vi "test_vision.vi"() -> ()   [LabVIEW 2011]
uses:
  <vilib>/vision/NI_Vision_Development_Module.lvlib
panel:
  out "Exe Times":u32[](array[numeric])
  out "Total Execution Time":u32
  out "Avg Execution Time":dbl
  in  "Range":cluster{"Lower value":sgl, "Upper value":sgl}={"Lower value"=218.04347, "Upper value"=255.0} {"Lower value" scale=0.0..255.0; "Upper value" scale=0.0..255.0}
  in  "Score Limits":T1={"Rect Coverage"=76.0, "Aspect Ratio"=0.0, "X Edge Strength"=40.0, "Y Edge Strength"=50.0}
  in  "Area Size Limit":i32=444
  in  "Particle Count Limit":i32=8
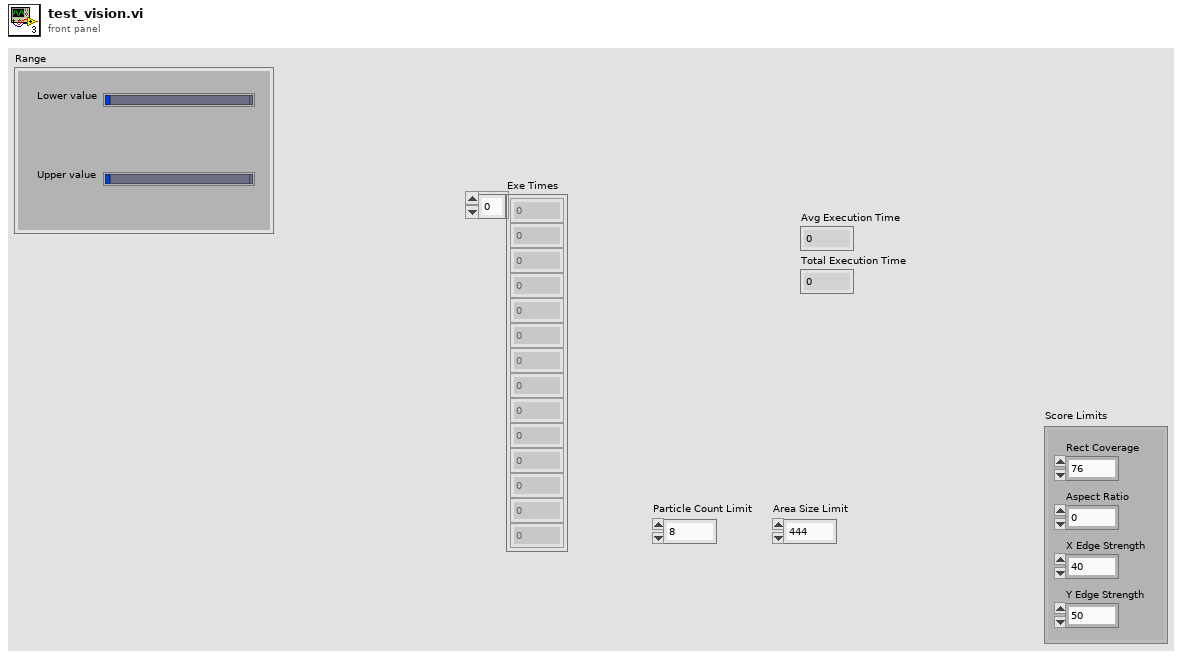
[diagram p1: front panel]
types:
  T1 = cluster{"Rect Coverage":dbl, "Aspect Ratio":dbl, "X Edge Strength":dbl, "Y Edge Strength":dbl}
  T2 = typedef "Image Type" = u32
  T3 = typedef "IMAQ Image.ctl" = refnum<image>
  T4 = enum32{"AutoM", "Close", "Dilate", "Erode", "Gradient", "Gradient in", "Gradient out", "HitMiss", "Open", "PClose", "POpen", "Thick", "Thin"}
  T5 = enum32{"AutoM", "Close", "Dilate", "Erode", "Gradient", "Gradient out", "Gradient in", "Hit miss", "Open", "PClose", "POpen", "Thick", "Thin"}
  T6 = cluster{cluster{"Left":dbl, "Top":dbl, "Right":dbl, "Bottom":dbl}, cluster{"Score":dbl, "Score":dbl, "X Score":dbl, "Y Score":dbl}, "Clipped Edge":cluster{"Left":bool, "Top":bool, "Right":bool, "Bottom":bool}}[]
  T7 = typedef "Camera State.ctl" = enum16{"No Targets", "Low Confidence", "Medium Confidence", "High Confidence", "Camera Error"}
  T8 = cluster{"X Position":dbl, "Distance":dbl, "Camera State":T7}
  T9 = typedef "Diamond Target Output.ctl" = cluster{"Position":cluster{"X":dbl, "Y":dbl, "Distance":dbl}, "Est. Position":T10, "Target Confidence":T11}
  T10 = typedef "Rectangle Position.ctl" = enum16{"Unknown", "Top", "Right", "Left", "Bottom"}
  T11 = typedef "Target Confidence.ctl" = enum16{"Good", "Good-Clipped Y", "Marginal-Clipped X"}
  T12 = typedef "Line.ctl" = cluster{"First Point":cluster{"X":dbl, "Y":dbl, "Index":dbl}, "Second Point":cluster{"X":dbl, "Y":dbl, "Index":dbl}, "theta":dbl, "Direction":T13, "Line Confidence":T14}
  T13 = typedef "Direction.ctl" = enum16{"Rt", "Rt-Up", "Up", "Lt-Up", "Lt", "Lt-Dn", "Dn", "Rt-Dn", "Unknown"}
  T14 = typedef "Line Confidence.ctl" = enum16{"Good", "Bad"}
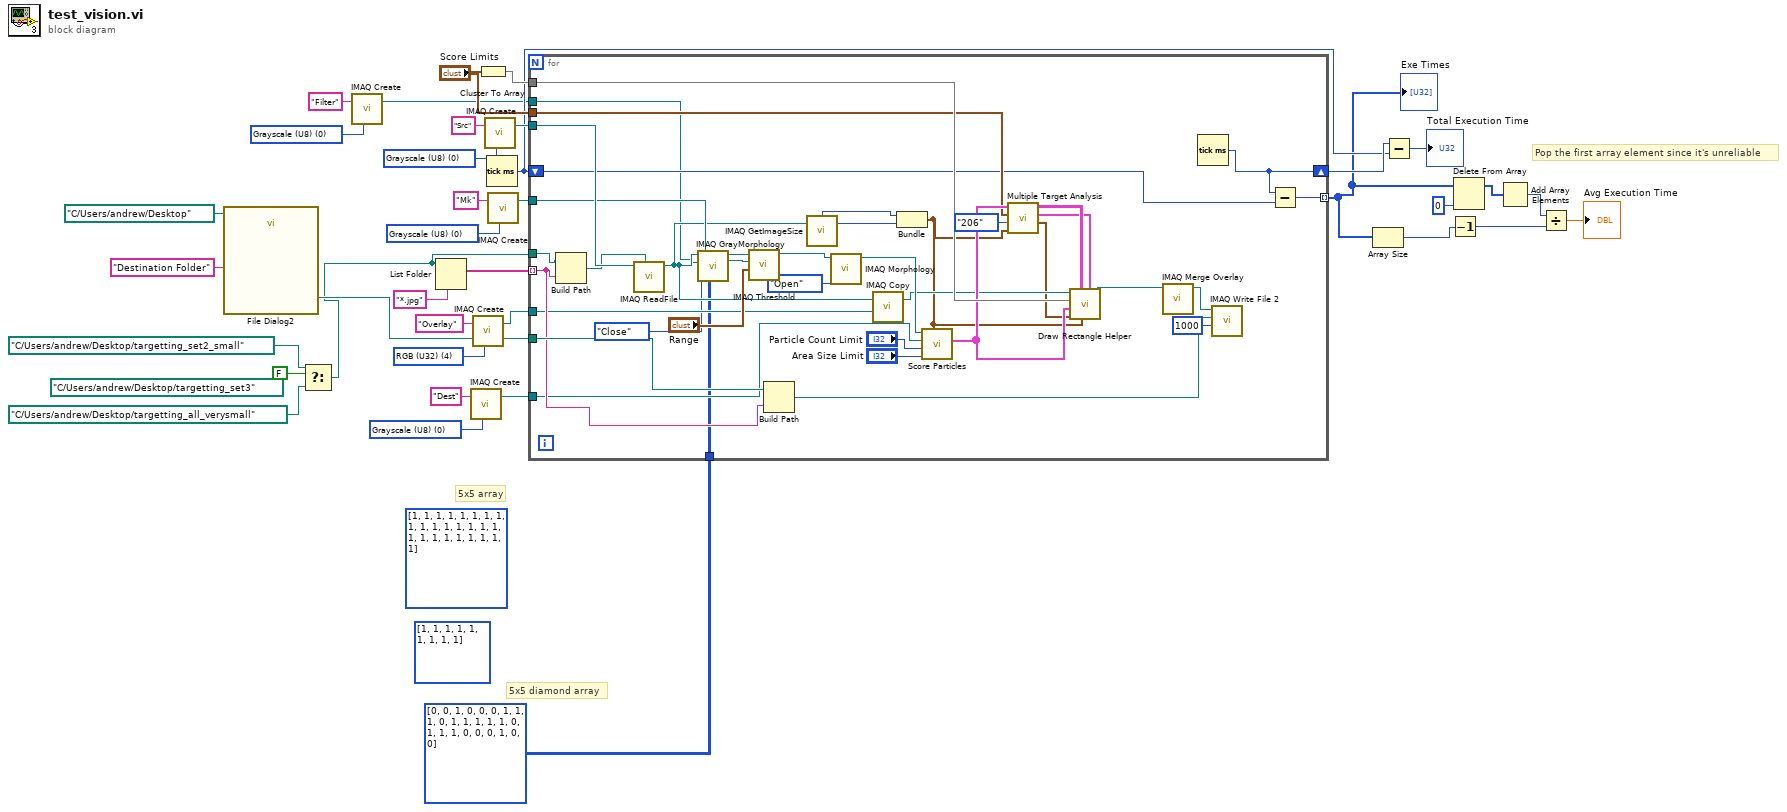
[diagram p0: block diagram]
diagram:
  (unwired) i32[][] [[1, 1, 1], [1, 1, 1], [1, 1, 1]] ("Structuring Element")
  (unwired) i32[][] [[1, 1, 1, 1, 1], [1, 1, 1, 1, 1], [1, 1, 1, 1, 1], [1, 1, 1, 1, 1], [1, 1, 1, 1, 1]] ("Structuring Element")
  w4 = T2 0 items=["Grayscale (U8)", "Grayscale (I16)", "Grayscale (SGL)", "Complex (CSG)", "RGB (U32)", "HSL (U32)", "RGB (U64)", "Grayscale (U16)"] ("Image Type")
  w17 = T2 4 items=["Grayscale (U8)", "Grayscale (I16)", "Grayscale (SGL)", "Complex (CSG)", "RGB (U32)", "HSL (U32)", "RGB (U64)", "Grayscale (U16)"] ("Image Type")
  (unwired) path "C:/Users/andrew/Desktop/targetting_set3" ("path")
  w23 = T2 0 items=["Grayscale (U8)", "Grayscale (I16)", "Grayscale (SGL)", "Complex (CSG)", "RGB (U32)", "HSL (U32)", "RGB (U64)", "Grayscale (U16)"] ("Image Type")
  w31 = T2 0 items=["Grayscale (U8)", "Grayscale (I16)", "Grayscale (SGL)", "Complex (CSG)", "RGB (U32)", "HSL (U32)", "RGB (U64)", "Grayscale (U16)"] ("Image Type")
  w33 = T2 0 items=["Grayscale (U8)", "Grayscale (I16)", "Grayscale (SGL)", "Complex (CSG)", "RGB (U32)", "HSL (U32)", "RGB (U64)", "Grayscale (U16)"] ("Image Type")
  # "5x5 diamond array"
  # "5x5 array"
  # "Pop the first array element since it's unreliable"
  n1 = call "File Dialog2"("start path"=path "C:/Users/andrew/Desktop", "prompt"="Destination Folder") -> ("selected path"=w27:path)  [unwired: 10 in, 3 out]
  n2 = Select(t=path "C:/Users/andrew/Desktop/targetting_set2_small" ("path"), s=FALSE, f=path "C:/Users/andrew/Desktop/targetting_all_verysmall" ("path")) -> (s? t:f=w20:path)
  n3 = call "IMAQ Create"("Image Name"="Filter", "Image Type"=w4) -> ("New Image"=w3:T3)  [unwired: 3 in, 1 out]
  n4 = List Folder(path=w20, pattern="*.jpg") -> (filenames=w35:string[])  [unwired: 2 in, 3 out]
  n5 = call "IMAQ Create"("Image Name"="Dest", "Image Type"=w23) -> ("New Image"=w24:T3)  [unwired: 3 in, 1 out]
  n6 = call "IMAQ Create"("Image Name"="Overlay", "Image Type"=w17) -> ("New Image"=w16:T3)  [unwired: 3 in, 1 out]
  n7 = Cluster To Array(cluster="Score Limits") -> (array=w28:dbl[])
  n8 = call "IMAQ Create"("Image Name"="Src", "Image Type"=w33) -> ("New Image"=w30:T3)  [unwired: 3 in, 1 out]
  n9 = Tick Count (ms)() -> (millisecond timer value=w12:u32)
  n10 = call "IMAQ Create"("Image Name"="Mk", "Image Type"=w31) -> ("New Image"=w29:T3)  [unwired: 3 in, 1 out]
  n11 = for {
    tunnel: w35 -> [w59] mode=indexing
    tunnel: w30 -> [w74]
    tunnel: w20 -> [w72]
    tunnel: w29 -> [w71]
    tunnel: w28 -> [w61]
    tunnel: w27 -> [w60]
    tunnel: w24 -> [w58]
    tunnel: "Score Limits" -> [w56]
    tunnel: w16 -> [w49]
    shift-right: [w45] -> w13
    shift-left: w12 -> [w44]
    tunnel: [w43] -> w10 mode=indexing
    tunnel: w3 -> [w40]
    tunnel: i32[][] [[0, 0, 1, 0, 0], [0, 1, 1, 1, 0], [1, 1, 1, 1, 1], [0, 1, 1, 1, 0], [0, 0, 1, 0, 0]] ("Structuring Element") -> [w38]
    n12 = Build Path(base path=w72, name or relative path=w59) -> (appended path=w73:path)
    n13 = call "IMAQ ReadFile"("File Path"=w73, "Image"=w74) -> ("Image Out"=w41:T3)  [unwired: 5 in, 4 out]
    n14 = call "IMAQ GrayMorphology"("Structuring Element"=w38, "Operation"=T4."Close", "Image Dst"=w40, "Image Src"=w41) -> ("Image Dst Out"=w42:T3)  [unwired: 6 in, 1 out]
    n15 = call "IMAQ Threshold"("Range"="Range", "Image Dst"=w71, "Image Src"=w42) -> ("Image Dst Out"=w70:T3)  [unwired: 7 in, 1 out]
    n16 = Build Path(base path=w60, name or relative path=w59) -> (appended path=w65:path)
    n17 = call "IMAQ GetImageSize"("Image"=w41) -> ("Y Resolution"=w50:i32, "X Resolution"=w51:i32)  [unwired: 3 in, 1 out]
    n18 = call "IMAQ Morphology"("Operation"=T5."Open", "Image Src"=w70) -> ("Image Dst Out"=w66:T3)  [unwired: 8 in, 1 out]
    n19 = call "IMAQ Copy"("Image Dst"=w49, "Image Src"=w41) -> ("Image Dst Out"=w48:T3)  [unwired: 4 in, 1 out]
    n20 = Bundle("X Resolution"=w51, "Y Resolution"=w50) -> (w46:cluster{"X Resolution":i32, "Y Resolution":i32})  [unwired: 1 in]
    n21 = call "Score Particles.vi"("Image Size"=w46, "Area Size Limit"="Area Size Limit", "Particle Count Limit"="Particle Count Limit", "Image Dst"=w58, "Image Refnum in"=w66) -> ("Targets"=w57:T6)  [unwired: 5 in, 1 out]
    n22 = call "Multiple Target Analysis.vi"("Image Size"=w46, "Camera Type"=enum16{"206", "1011"}."206", "Score Limits"=w56, "Targets"=w57) -> ("Targetting Output"=w47:T8, "Diamond Targets"=w53:T9[], "Lines"=w54:T12[][])  [unwired: 5 in]
    n23 = call "Draw Rectangle Helper.vi"("Diamond Targets"=w53, "Image Size"=w46, "Lines"=w54, "Targetting Output"=w47, "Targets"=w57, "Score Limits"=w61, "Refnum in"=w48) -> ("Refnum out"=w63:T3)  [unwired: 4 in]
    n24 = call "IMAQ Merge Overlay"("Image Src"=w63) -> ("Image Dst Out"=w62:T3)  [unwired: 9 in, 1 out]
    n25 = Tick Count (ms)() -> (millisecond timer value=w45:u32)
    n26 = call-poly "IMAQ Write File 2"("Image Quality"=u32 1000, "File Path"=w65, "Image"=w62) -> ()  [unwired: 7 in, 2 out]
    n27 = Subtract(x=w45, y=w44) -> (x-y=w43:u32)
  }
  "Exe Times" <- w10
  n28 = Array Size(array=w10) -> (size(s)=w7:i32)
  n29 = Subtract(x=w13, y=w12) -> (x-y=→"Total Execution Time":u32)
  n30 = Decrement(x=w7) -> (x-1=w6:i32)
  n31 = Delete From Array(array=w10, index=0) -> (array with subset deleted=w9:u32[])  [unwired: 1 in, 1 out]
  n32 = Add Array Elements(numeric array=w9) -> (sum=w15:u32)
  n33 = Divide(x=w15, y=w6) -> (x/y=→"Avg Execution Time":dbl)
